vi "cont.vi"() -> ()   [LabVIEW 2013]
panel:
  in  "Numeric":u16=100
  out "Adc 2":dbl(graph)
  out "Adc 1":dbl(graph)
  out "Error out":errorcluster
  out "VISA resource name out":refnum<visa-resource-name>
  in  "stop":bool
  in  "VISA resource name":refnum<visa-resource-name>="ASRL2::INSTR"
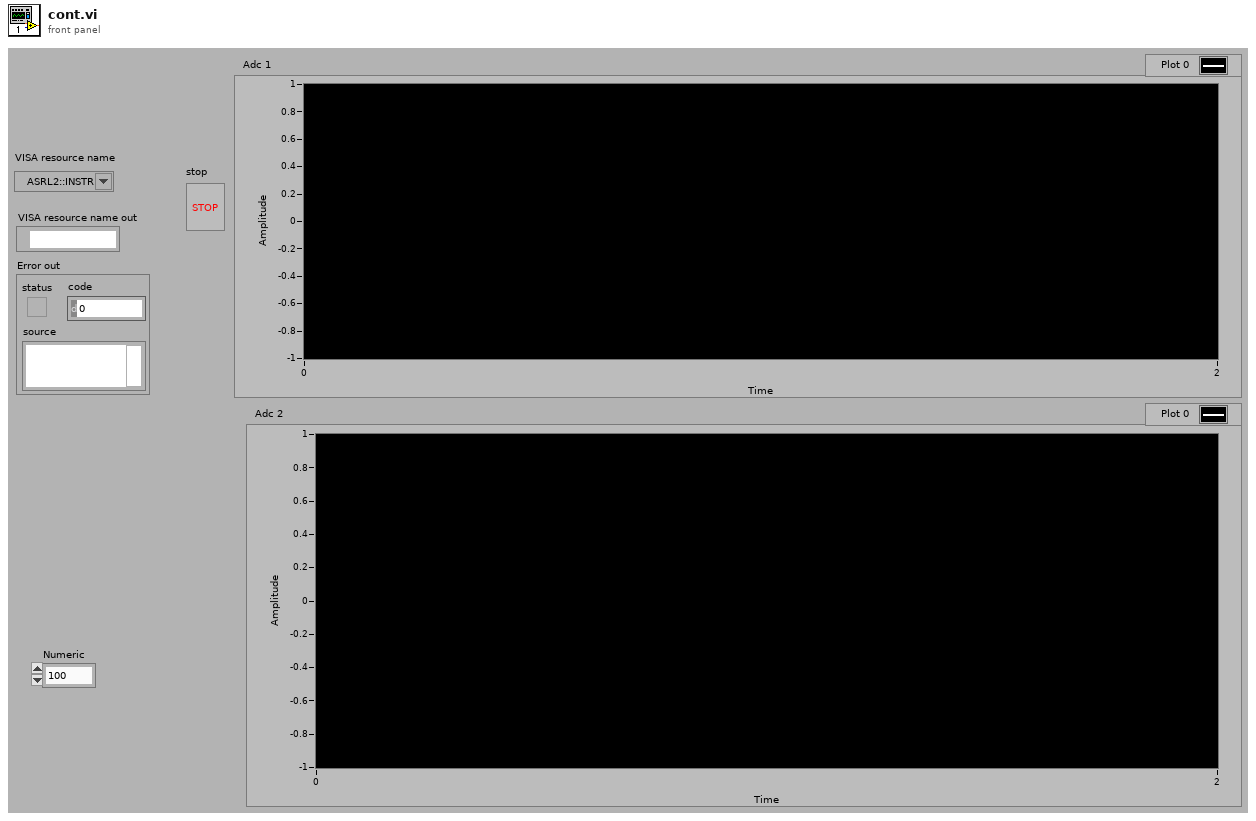
[diagram p1: front panel]
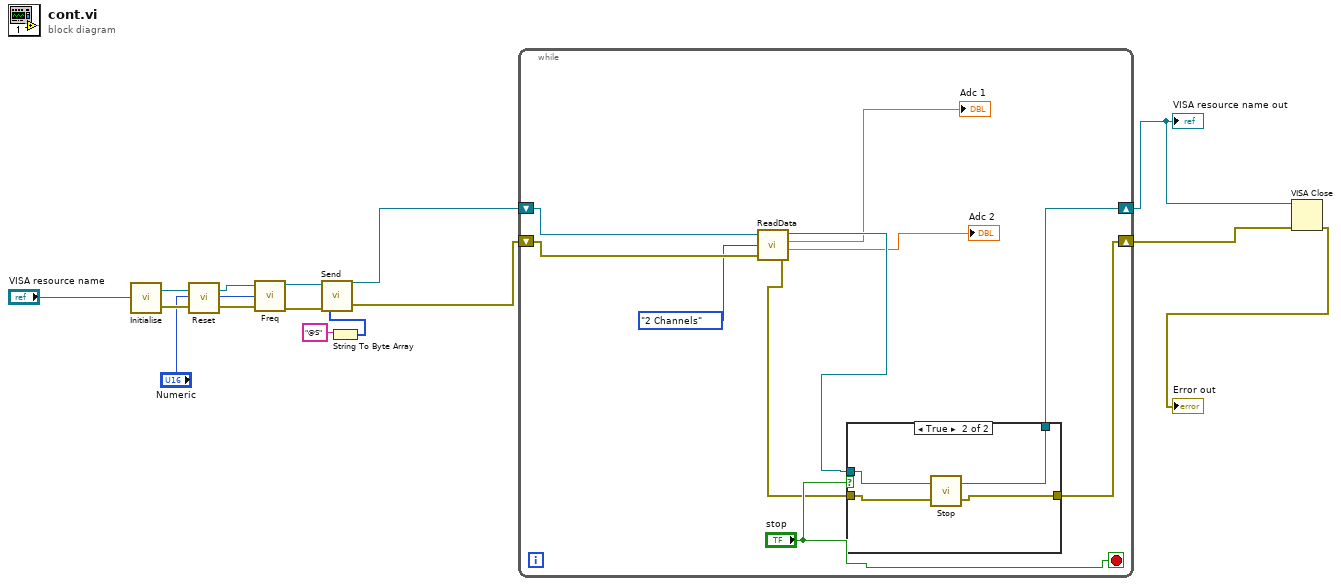
[diagram p0: block diagram]
diagram:
  n1 = call "Initialise.vi"("VISA resource name"="VISA resource name") -> ("Duplicate VISA resource name"=w14:refnum<visa-resource-name>, "Error out"=w13:errorcluster)
  n2 = call "Reset.vi"("error in (no error)"=w13, "VISA resource name"=w14) -> ("Error out"=w3:errorcluster, "Duplicate VISA resource name"=w5:refnum<visa-resource-name>)
  n3 = call "Freq.vi"("VISA resource name"=w5, "Numeric"="Numeric", "Error in (no error)"=w3) -> ("VISA resource name out"=w4:refnum<visa-resource-name>, "Error out"=w2:errorcluster)  [unwired: 2 in]
  n4 = String To Byte Array(string="@S") -> (unsigned byte array=w8:u8[])
  n5 = call "Send.vi"("Error in (no error)"=w2, "Bytes to send"=w8, "VISA resource name"=w4) -> ("Error out"=w6:errorcluster, "VISA resource name out"=w7:refnum<visa-resource-name>)
  n6 = while {
    shift-right: [w22] -> w12
    shift-left: w7 -> [w18]
    shift-right: [w24] -> w11
    shift-left: w6 -> [w17]
    stop <- "stop" stop-if-true
    n7 = call "ReadData.vi"("VISA resource name"=w18, "Number of channels"=enum16{"1 Channel", "2 Channels"}."2 Channels", "Error in (no error)"=w17) -> ("VISA resource name out"=w21:refnum<visa-resource-name>, "Adc 1"=→"Adc 1":dbl, "Adc 2"=→"Adc 2":dbl, "Error out"=w23:errorcluster)
    n8 = case shown="True" "stop" {
      tunnel: w21 -> [w27 w31]
      tunnel: w23 -> [w26 w30]
      tunnel: [w27 w29] -> w22
      tunnel: [w26 w28] -> w24
      frame False {
      }
      frame True {
        n9 = call "Stop.vi"("Error in (no error)"=w30, "VISA resource name"=w31) -> ("Error out"=w28:errorcluster, "VISA resource name out"=w29:refnum<visa-resource-name>)
      }
    }
  }
  "VISA resource name out" <- w12
  n10 = VISA Close(VISA resource name=w12, error in (no error)=w11) -> (error out=→"Error out":errorcluster)
